vi "FlatToRichGreeter_res.vi"(5 "OutputClusterType":T1, 11 "InputCluster":T2) -> (3 "OutputCluster":T1)   [LabVIEW 2019, in "Generated_server.lvlib"]
uses:
  Generated_server.lvlib
  Greeter_res_Flat.ctl
  Greeter_res.ctl
  Greeter_res_res_oneof/Greeter_res_res_oneof.lvclass
  Greeter_res_res_oneof/Greeter_res_res_oneof.lvclass/Greeter_res_res_oneof.ctl
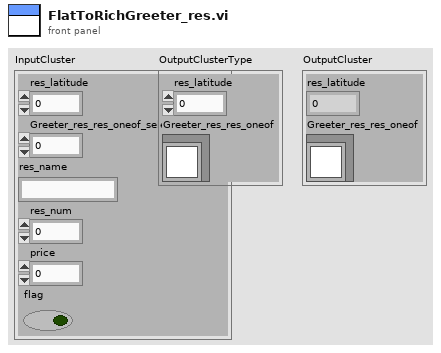
[diagram p1: front panel]
types:
  T1 = typedef "Generated_server.lvlib/Greeter_res.ctl" = cluster{"res_latitude":i32, "Greeter_res_res_oneof":refnum<class "Greeter_res_res_oneof.lvclass">}
  T2 = typedef "Generated_server.lvlib/Greeter_res_Flat.ctl" = cluster{"res_latitude":i32, "Greeter_res_res_oneof_selected_index":i32, "res_name":string, "res_num":i32, "price":sgl, "flag":bool}
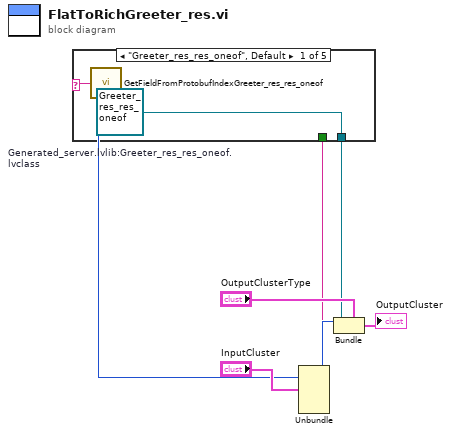
[diagram p0: block diagram]
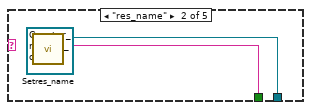
[diagram p2: hidden frame]
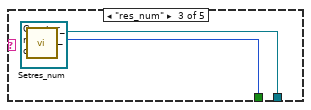
[diagram p3: hidden frame]
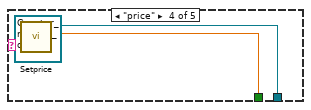
[diagram p4: hidden frame]
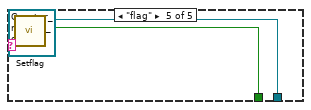
[diagram p5: hidden frame]
diagram:
  n1 = Unbundle "Unbundle"("InputCluster") -> ("res_latitude"=w8:i32, "Greeter_res_res_oneof_selected_index"=w7:i32, "res_name"=w4:string, "res_num"=w3:i32, "price"=w2:sgl, "flag"=w1:bool)
  n2 = call "GetFieldFromProtobufIndexGreeter_res_res_oneof.vi"("protobuf index"=w7) -> ("oneof field name"=w6:string)
  n3 = case "Greeter_res_res_oneof" shown="\"Greeter_res_res_oneof\", Default" w6 {
    tunnel: [w12 w14 w17 w20 w23] -> w5
    tunnel: w4 -> [_ w15 _ _ _]
    tunnel: w3 -> [_ _ w18 _ _]
    tunnel: w2 -> [_ _ _ w21 _]
    tunnel: w1 -> [_ _ _ _ w24]
    frame "Greeter_res_res_oneof", Default {
      w12 = refnum<class "Greeter_res_res_oneof.lvclass"> refnum  # Generated_server.lvlib:Greeter_res_res_oneof.lvclass
    }
    frame "res_name" {
      n4 = call "Setres_name.vi"("Set_Val"=w15, "OneOfTemplate in"=refnum<class "Greeter_res_res_oneof.lvclass"> refnum) -> ("OneOfTemplate out"=w14:refnum<class "Greeter_res_res_oneof.lvclass">)  [unwired: 8 in, 1 out]
    }
    frame "res_num" {
      n5 = call "Setres_num.vi"("Set_Val"=w18, "OneOfTemplate in"=refnum<class "Greeter_res_res_oneof.lvclass"> refnum) -> ("OneOfTemplate out"=w17:refnum<class "Greeter_res_res_oneof.lvclass">)  [unwired: 8 in, 1 out]
    }
    frame "price" {
      n6 = call "Setprice.vi"("Set_Val"=w21, "OneOfTemplate in"=refnum<class "Greeter_res_res_oneof.lvclass"> refnum) -> ("OneOfTemplate out"=w20:refnum<class "Greeter_res_res_oneof.lvclass">)  [unwired: 8 in, 1 out]
    }
    frame "flag" {
      n7 = call "Setflag.vi"("Set_Val"=w24, "OneOfTemplate in"=refnum<class "Greeter_res_res_oneof.lvclass"> refnum) -> ("OneOfTemplate out"=w23:refnum<class "Greeter_res_res_oneof.lvclass">)  [unwired: 8 in, 1 out]
    }
  }
  n8 = Bundle "Bundle"(cluster="OutputClusterType", "res_latitude"=w8, "Greeter_res_res_oneof"=w5) -> (→"OutputCluster":T1)
